vi "Name.vi"(11 "EStop Source in":refnum<class "EStop Source.lvclass">) -> (2 "Name":string)   [LabVIEW 2020, in "VolatusControl.lvlib" / "EStop Source.lvclass"]
uses:
  EStop Source.lvclass
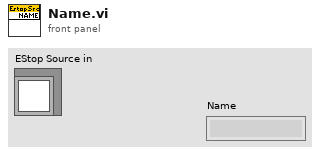
[diagram p1: front panel]
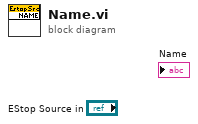
[diagram p0: block diagram]
diagram:
